vi "CAEN_HVSystem.get data to modify.vi"(0 "i ref in":refnum<vi>, 3 "ms timeout (10000)":i32=10000, 5 "error in (no error)":errorcluster) -> (14 "i ref out":refnum<vi>, 16 "i attribute":T1 {"FrontPanOut"."FrontPanOut" format="%.0b"; "FrontPanIn"."FrontPanIn" format="%.0b"; "GenSignCfg"."GenSignCfg" format="%.0b"}, 17 "timed out":bool, 19 "error out":errorcluster)   [LabVIEW 2014, in "CAEN_HVSystem.lvlib"]
doc: "Reads the attribute data of the object after the access to the data has been locked by the \"acquire\" method. If the attribute data has been locked already, this methods waits until the attribute data is unlocked or there is a timeout.\n\nThe attribute data must be unlocked using the methods \"release\" or \"set modified data\".\n\nLicense Agreement for this software:\n\nCopyright (C)\nGesellschaft für Schwerionenforschung, GSI\nPlanckstr. 1\n64291 Darmstadt\nGermany\n\nContact: D.Beck@gsi.de \n\nThis program is free software; you can redistribute it and/or modify it under the terms of the GNU General Public License as published by the Free Software Foundation; either version 2 of the license, or (at your option) any later version.\n\nThis program is distributed in the hope that it will be useful, but WITHOUT ANY WARRANTY; without even the implied warranty of MERCHANTABILITY or FITNESS FOR A PARTICULAR PURPOSE. See the GNU General License for more details (http://www.gnu.org).\n\nGesellschaft für Schwerionenforschung, GSI\nPlanckstr. 1, 64291 Darmstadt, Germany\nFor all questions and ideas contact: M.Richter@gsi.de, H.Brand@gsi.de or D.Beck@gsi.de.\nLast update: 17-JUN-2004"
uses:
  CAEN_HVSystem.lvlib
  CAEN_HVSystem.i attribute.ctl
  CS_Core/CSObj/CSObj.lvlib
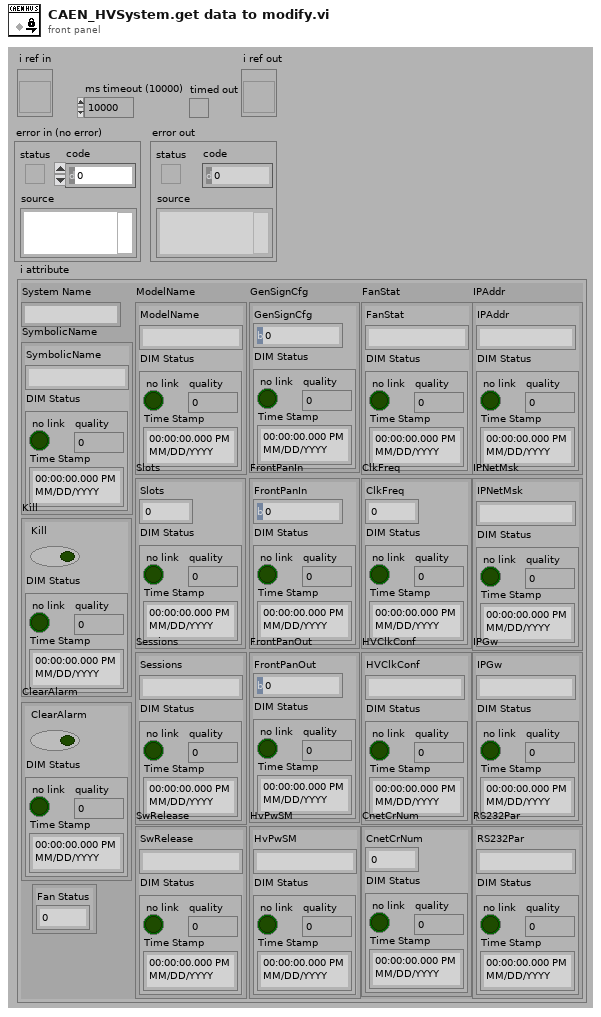
[diagram p1: front panel]
types:
  T1 = typedef "CAEN_HVSystem.lvlib/CAEN_HVSystem.i attribute.ctl" = cluster{"System Name":string, "DIM Service IDs":cluster{"Fan Status":i32}, "SymbolicName":cluster{"SymbolicName":string, "DIM Status":cluster{"no link":bool, "quality":i32, "Time Stamp":timestamp}}, "ModelName":cluster{"ModelName":string, "DIM Status":cluster{"no link":bool, "quality":i32, "Time Stamp":timestamp}}, "Slots":cluster{"Slots":i16, "DIM Status":cluster{"no link":bool, "quality":i32, "Time Stamp":timestamp}}, "Kill":cluster{"Kill":bool, "DIM Status":cluster{"no link":bool, "quality":i32, "Time Stamp":timestamp}}, "ClearAlarm":cluster{"ClearAlarm":bool, "DIM Status":cluster{"no link":bool, "quality":i32, "Time Stamp":timestamp}}, "Sessions":cluster{"Sessions":string, "DIM Status":cluster{"no link":bool, "quality":i32, "Time Stamp":timestamp}}, "SwRelease":cluster{"SwRelease":string, "DIM Status":cluster{"no link":bool, "quality":i32, "Time Stamp":timestamp}}, "GenSignCfg":cluster{"GenSignCfg":i16, "DIM Status":cluster{"no link":bool, "quality":i32, "Time Stamp":timestamp}}, "FrontPanIn":cluster{"FrontPanIn":i16, "DIM Status":cluster{"no link":bool, "quality":i32, "Time Stamp":timestamp}}, "FrontPanOut":cluster{"FrontPanOut":i16, "DIM Status":cluster{"no link":bool, "quality":i32, "Time Stamp":timestamp}}, "HvPwSM":cluster{"HvPwSM":string, "DIM Status":cluster{"no link":bool, "quality":i32, "Time Stamp":timestamp}}, "FanStat":cluster{"FanStat":string, "DIM Status":cluster{"no link":bool, "quality":i32, "Time Stamp":timestamp}}, "ClkFreq":cluster{"ClkFreq":i16, "DIM Status":cluster{"no link":bool, "quality":i32, "Time Stamp":timestamp}}, "HVClkConf":cluster{"HVClkConf":string, "DIM Status":cluster{"no link":bool, "quality":i32, "Time Stamp":timestamp}}, "CnetCrNum":cluster{"CnetCrNum":i16, "DIM Status":cluster{"no link":bool, "quality":i32, "Time Stamp":timestamp}}, "IPAddr":cluster{"IPAddr":string, "DIM Status":cluster{"no link":bool, "quality":i32, "Time Stamp":timestamp}}, "IPNetMsk":cluster{"IPNetMsk":string, "DIM Status":cluster{"no link":bool, "quality":i32, "Time Stamp":timestamp}}, "IPGw":cluster{"IPGw":string, "DIM Status":cluster{"no link":bool, "quality":i32, "Time Stamp":timestamp}}, "RS232Par":cluster{"RS232Par":string, "DIM Status":cluster{"no link":bool, "quality":i32, "Time Stamp":timestamp}}}
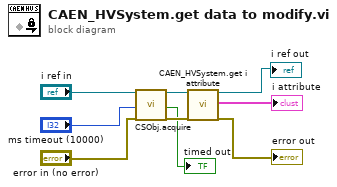
[diagram p0: block diagram]
diagram:
  n1 = call "CSObj.acquire.vi"("i ref in"="i ref in", "ms timeout (10000)"="ms timeout (10000)", "error in (no error)"="error in (no error)") -> ("i ref out"=w8:refnum<vi>, "timed out"=→"timed out":bool, "error out"=w5:errorcluster)  [unwired: 14 in]
  n2 = call "CAEN_HVSystem.get i attribute.vi"("i ref in"=w8, "error in (no error)"=w5) -> ("i ref out"=→"i ref out":refnum<vi>, "i attribute"=→"i attribute":T1, "error out"=→"error out":errorcluster)  [unwired: 15 in]
